vi "FPGA.vi"() -> ()   [LabVIEW 2013]
doc: "This is the primary FPGA VI for the Build Your Own Embedded System project."
uses:
  <vilib>/Platform/TimedLoop/XDataNode/timing_clust.ctl
  <vilib>/Platform/TimedLoop/XDataNode/nitl_modes.ctl
  <vilib>/Platform/TimedLoop/XDataNode/wakeup.ctl
  <vilib>/rvi/FXPMathLib/FxpDiv/subVIs/nifxpmath_Div_SimConfig.ctl
  <vilib>/rvi/Emulation/niFpgaSctlEmulationGetInTimedLoop.vi
  <vilib>/rvi/Emulation/niFpgaEmulationReportErrorSimple.vi
  <vilib>/rvi/Emulation/niFpgaGetClockAttributes.vi
  <vilib>/rvi/eio/common/nirviEmuTemplateMethod_errors.vi
  <vilib>/rvi/Emulation/niFpgaCriticalErrorInLSC.vi
  <vilib>/rvi/Analysis/utilities/niFPGA Threshold Crossing Logic.vi
  <vilib>/rvi/FXPMathLib/FxpDiv/simVIs/DllFxpDivTemp_sub.vi
  <vilib>/rvi/Analysis/measure/period/templates/niFPGA Period Edge Direction.ctl
  <vilib>/eio/EIONode/EIONode.xnode
  <vilib>/rvi/Analysis/measure/period/XNode/niFpgaAnalogPeriod.xnode
  <vilib>/Platform/TimedLoop/XDataNode/XDataNode.xnode
  <vilib>/rvi/FXPMathLib/FxpDiv/XNode/nifxpmath_Div.xnode
  <vilib>/rvi/Analysis/measure/butterworth/XNode/niFpgaButterworthFilter.xnode
  <vilib>/addons/control/pid/fpga.llb/XNode/niFpgaPID.xnode
  <vilib>/rvi/FXPMathLib/FxpInterpret/XNode/nifxpmath_Interpret.xnode
  <vilib>/Platform/TimedLoop/XDataNode/XDNodeRunTimeDep.lvlib
panel:
  in  "Invert Polarity?":bool=TRUE
  in  "stop bits (10: 1 bit)":u16(ring)=10 items=["1.0"=10, "1.5"=15, "2.0"=20]
  in  "data bits (8)":i32=8 min=5 max=8 step=1
  in  "parity (0:none)":enum16{"None", "Odd", "Even", "Mark", "Space"}(ring)
  in  "baud rate":u32=1200000
  out "PIDOut":fxp<+/-,16,8>
  in  "PIDSetpoint":fxp<+/-,16,18>
  in  "PID gains":T1={"proportional gain (Kc)"=1.0, "integral gain (Kc*Ts/Ti)"=0.015625, "derivative gain (Kc*Td/Ts)"=0.0}
  in  "CommandFilterCoeff":i32[](array[numeric])=[-955995012, 2025731616, 1001305, -1023351008, 2092954700, 1034533]
  in  "UsePID":bool
  in  "DeadCount":u32=100
  in  "JerkThresh":fxp<+/-,37,22>=100.0
  out "Jerk":fxp<+/-,37,22>
  out "Accel":fxp<+/-,33,18>
  out "Speed":fxp<+/-,33,18>
  out "State":enum16{"Forward", "Reverse"}(ring)
  out "FilteredRPM":fxp<+/-,33,18>
  out "Direction":bool
  in  "SpeedFilterCoeff":i32[](array[numeric])=[-955995012, 2025731616, 1001305, -1023351008, 2092954700, 1034533]
  out "SpeedCommandOut":fxp<+/-,23,8>
  in  "PeriodHysteresis":fxp<+,23,4>=0.5
  in  "PeriodThreshold":fxp<+/-,24,5>=2.0
  in  "SpeedCommand":fxp<+/-,20,5>
  in  "DriveEnable":bool
  out "Potentiometer":fxp<+/-,24,5>
  out "RPM":fxp<+,32,16>
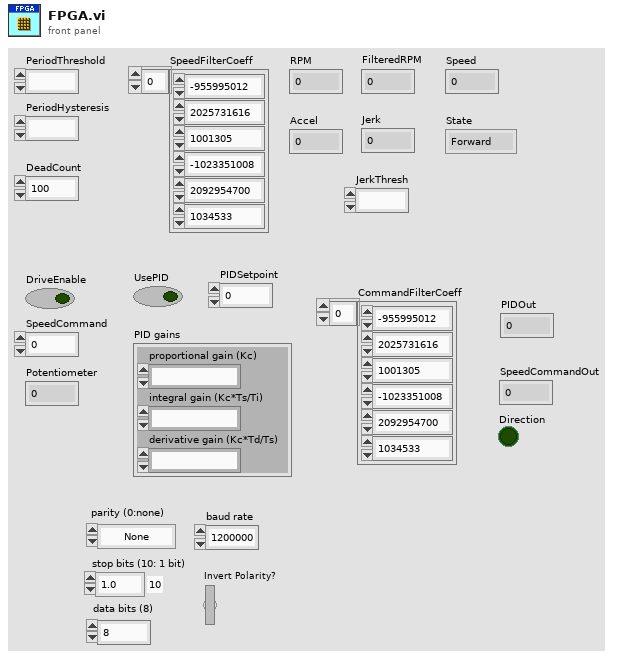
[diagram p1: front panel]
types:
  T1 = cluster{"proportional gain (Kc)":fxp<+/-,16,8>, "integral gain (Kc*Ts/Ti)":fxp<+/-,16,8>, "derivative gain (Kc*Td/Ts)":fxp<+/-,16,8>}
  T2 = typedef "XDNodeRunTimeDep.lvlib/timing_clust.ctl" = cluster{"Expected End [f-1]":u64, "Actual End [f-1]":u64, "Finished Late? [f-1]":bool, "Expected End [i-1]":u64, "Actual End [i-1]":u64, "Finished Late? [i-1]":bool, "Expected Start [i]":u64, "Actual Start [i]":u64, "Expected Start [f]":u64, "Actual Start [f]":u64, "Source Name":string, "Structure Name":string, "Period":i64, "Deadline":i64, "Offset":i64, "Start":i64, "Priority":i32, "Timeout":i32, "Mode":T3, "Wakeup Reason":T4, "Error":errorcluster, "Source Type":string, "Secondary Source Type":string, "Global End Time":u64, "Global Start Time":u64, "Frame Duration":u64, "Iteration Duration":u64, "Assigned CPU":i32, "I/O Scan Engine Mode":u32}
  T3 = typedef "XDNodeRunTimeDep.lvlib/nitl_modes.ctl" = enum32{"No Change", "Process missed periods, maintain original phase", "Discard missed periods, maintain original phase", "Process missed periods, ignore original phase", "Discard missed periods, ignore original phase"}
  T4 = typedef "XDNodeRunTimeDep.lvlib/wakeup.ctl" = enum32{"Normal", "Aborted", "Asynchronous wakeup", "Timing source error", "Timed loop error", "Timeout"}
  T5 = cluster{"proportional gain (Kc)":i16, "integral gain (Kc*Ts/Ti)":i16, "derivative gain (Kc*Td/Ts)":i16}
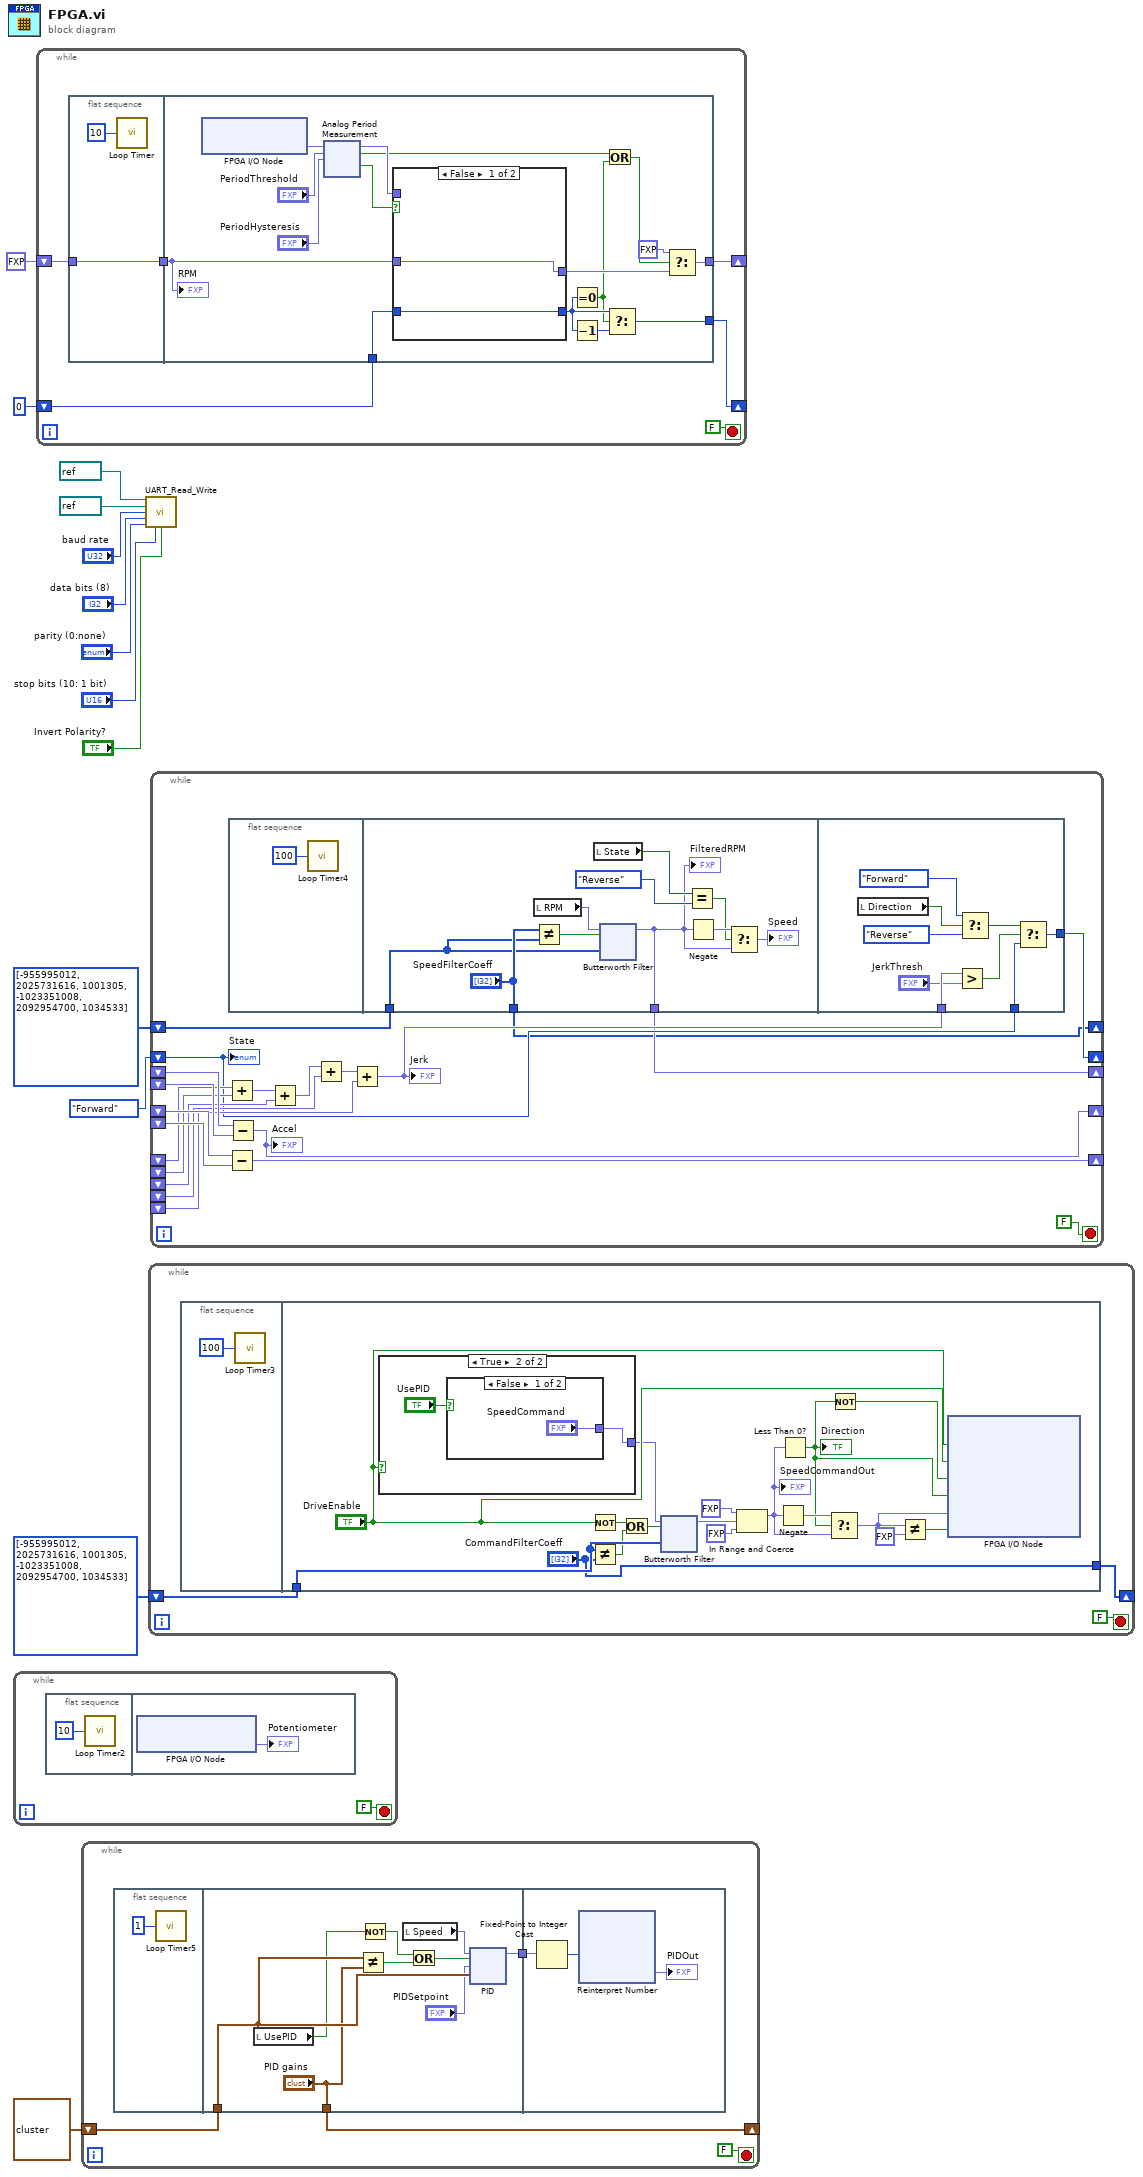
[diagram p0: block diagram]
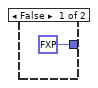
[diagram p2: hidden frame]
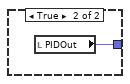
[diagram p3: hidden frame]
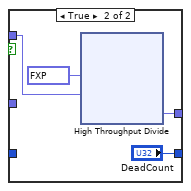
[diagram p4: hidden frame]
diagram:
  n1 = while {
    stop <- FALSE stop-if-true
    n2 = flat-sequence {
      frame #0 {
        n3 = call "Loop Timer2"("Count(mSec)"=u32 10 ("Count(uSec)")) -> ()  [unwired: 1 out]
      }
      frame #1 {
        n4 = xnode "FPGA I/O Node"() -> ("Potentiometer"=→"Potentiometer":fxp<+/-,24,5>)  [unwired: 1 in, 1 out]
      }
    }
  }
  n5 = while {
    shift-right: [w21] -> _
    shift-left: fxp<+,32,16> 0.0 ("x/y") -> [w20]
    shift-right: [w18] -> _
    shift-left: u32 0 ("DeadCount") -> [w17]
    stop <- FALSE stop-if-true
    n6 = flat-sequence {
      tunnel: w20 -> [w24]
      tunnel: [w24] -> w19
      tunnel: w19 -> [w31]
      tunnel: [w34] -> w21
      tunnel: [w27] -> w18
      tunnel: w17 -> [w32]
      frame #0 {
        n7 = call "Loop Timer"("Count(uSec)"=u32 10) -> ()  [unwired: 1 out]
      }
      frame #1 {
        n8 = xnode "FPGA I/O Node"() -> ("MotorPWM"=w40:fxp<+/-,24,5>)  [unwired: 1 in, 1 out]
        n9 = xnode "Analog Period Measurement"("input data"=w40, "threshold level"="PeriodThreshold", "hysteresis"="PeriodHysteresis") -> ("period (samples)"=w38:fxp<+,32,16>, "output valid"=w39:bool, "timeout"=w30:bool)  [unwired: 2 in, 1 out]
        n10 = case shown="False" w39 {
          tunnel: w38 -> [_ w46]
          tunnel: [w42 w44] -> w35
          tunnel: w31 -> [w42 _]
          tunnel: [w41 "DeadCount"] -> w28
          tunnel: w32 -> [w41 _]
          frame False {
          }
          frame True {
            n11 = xnode "High Throughput Divide"("x"=fxp<+,32,32> 100000.0, "y"=w46) -> ("x/y"=w44:fxp<+,32,16>)
          }
        }
        n12 = Equal To 0?(x=w28) -> (x = 0?=w25:bool)
        n13 = Decrement(x=w28) -> (x-1=w26:u32)
        n14 = Or(x=w30, y=w25) -> (x .or. y?=w29:bool)
        n15 = Select(t=w28, s=w25, f=w26) -> (s? t:f=w27:u32)
        n16 = Select(t=fxp<+,32,16> 0.0, s=w29, f=w35) -> (s? t:f=w34:fxp<+,32,16>)
        "RPM" <- w31
      }
    }
  }
  n17 = while {
    shift-right: [w192] -> _
    shift-left: T1 {"proportional gain (Kc)"=1.0, "integral gain (Kc*Ts/Ti)"=0.015625, "derivative gain (Kc*Td/Ts)"=0.0} ("PID gains") -> [w191]
    stop <- FALSE stop-if-true
    n18 = flat-sequence {
      tunnel: ["PID gains"] -> w192
      tunnel: w191 -> [w202]
      tunnel: [w194] -> w190
      tunnel: w190 -> [w233]
      frame #0 {
        n19 = call "Loop Timer5"("Count(mSec)"=u32 1 ("Count(uSec)")) -> ()  [unwired: 1 out]
      }
      frame #1 {
        n20 = local read "UsePID"() -> (w200:bool)
        n21 = Not Equal?(x=w202, y="PID gains") -> (x != y?=w198:bool)
        n22 = Not(x=w200) -> (.not. x?=w199:bool)
        n23 = local read "Speed"() -> (w196:fxp<+/-,33,18>)
        n24 = Or(x=w199, y=w198) -> (x .or. y?=w197:bool)
        n25 = xnode "PID"("process variable"=w196, "reset?"=w197, "setpoint"="PIDSetpoint", "PID gains"=w202) -> ("output"=w194:fxp<+/-,16,18>)  [unwired: 1 in]
      }
      frame #2 {
        n26 = Fixed-Point to Integer Cast(1:w233) -> (0:w232:i16)
        n27 = xnode "Reinterpret Number"("x"=w232) -> ("y"=→"PIDOut":fxp<+/-,16,8>)
      }
    }
  }
  n28 = call "UART_Read_Write.vi"("Transmit"=refnum<k21> "TX", "Receive"=refnum<k21> "RX", "baud rate (9600)"="baud rate", "data bits (8)"="data bits (8)", "parity (0:none)"="parity (0:none)", "stop bits (10: 1 bit)"="stop bits (10: 1 bit)", "Invert Polarity?"="Invert Polarity?") -> ()  [unwired: 9 in]
  n29 = while {
    shift-right: [w235] -> _
    shift-left: i32[] [-955995012, 2025731616, 1001305, -1023351008, 2092954700, 1034533] ("CommandFilterCoeff") -> [w234]
    stop <- FALSE stop-if-true
    n30 = flat-sequence {
      tunnel: ["CommandFilterCoeff"] -> w235
      tunnel: w234 -> [w245]
      frame #0 {
        n31 = call "Loop Timer3"("Count(uSec)"=u32 100) -> ()  [unwired: 1 out]
      }
      frame #1 {
        n32 = case shown="True" "DriveEnable" {
          tunnel: [fxp<+/-,20,5> 0.0 ("SpeedCommand") w265] -> w240
          frame False {
          }
          frame True {
            n33 = case shown="False" "UsePID" {
              tunnel: ["SpeedCommand" w267] -> w265
              frame False {
              }
              frame True {
                n34 = local read "PIDOut"() -> (w267:fxp<+/-,16,8>)
              }
            }
          }
        }
        n35 = Not(x="DriveEnable") -> (.not. x?=w243:bool)
        n36 = Not Equal?(x=w245, y="CommandFilterCoeff") -> (x != y?=w242:bool)
        n37 = Or(x=w243, y=w242) -> (x .or. y?=w241:bool)
        n38 = xnode "Butterworth Filter"("input data"=w240, "reset"=w241, "scaled coefficients"=w245) -> ("output data"=w239:fxp<+/-,23,8>)
        n39 = In Range and Coerce(upper limit=fxp<+/-,20,5> 5.0, x=w239, lower limit=fxp<+/-,20,5> -5.0) -> (coerced(x)=w238:fxp<+/-,23,8>)  [unwired: 1 out]
        "SpeedCommandOut" <- w238
        n40 = Negate(x=w238) -> (-x=w251:fxp<+/-,20,5>)
        n41 = Less Than 0?(x=w238) -> (x < 0?=w247:bool)
        "Direction" <- w247
        n42 = Select(t=w251, s=w247, f=w238) -> (s? t:f=w250:fxp<+/-,23,8>)
        n43 = Not(x=w247) -> (.not. x?=w252:bool)
        n44 = Not Equal?(x=w250, y=fxp<+/-,20,5> 0.0) -> (x != y?=w253:bool)
        n45 = xnode "FPGA I/O Node"("EnableOut"="DriveEnable", "Enable"="DriveEnable", "DirectionOut"=w252, "Direction"=w247, "SpeedCommand"=w250, "Running"=w253) -> ()  [unwired: 6 in, 6 out]
      }
    }
  }
  n46 = while {
    shift-right: [w270] -> _
    shift-left: _ -> [w287]
    shift-right: [w271] -> _
    shift-left: enum16{"Forward", "Reverse"}."Forward" -> [w272]
    shift-left: _ -> [w286]
    shift-right: [w285] -> _
    shift-left: _ -> [w284]
    shift-left: _ -> [w283]
    shift-right: [w282] -> _
    shift-left: _ -> [w281]
    shift-left: _ -> [w280]
    shift-left: _ -> [w278]
    shift-left: _ -> [w276]
    shift-left: _ -> [w274]
    shift-right: [w269] -> _
    shift-left: i32[] [-955995012, 2025731616, 1001305, -1023351008, 2092954700, 1034533] ("FilterCoeff") -> [w268]
    stop <- FALSE stop-if-true
    n47 = Add(x=w281, y=w280) -> (x+y=w279:fxp<+/-,35,20>)
    n48 = Subtract(x=w284, y=w283) -> (x-y=w282:fxp<+/-,34,19>)
    n49 = Subtract(x=w287, y=w286) -> (x-y=w285:fxp<+/-,33,18>)
    "Accel" <- w285
    n50 = flat-sequence {
      tunnel: [w293] -> w270
      tunnel: ["SpeedFilterCoeff"] -> w269
      tunnel: w268 -> [w291]
      tunnel: w273 -> [w316]
      tunnel: w272 -> [w313]
      tunnel: [w312] -> w271
      frame #0 {
        n51 = call "Loop Timer4"("Count(uSec)"=u32 100) -> ()  [unwired: 1 out]
      }
      frame #1 {
        n52 = local read "RPM"() -> (w299:fxp<+,32,16>)
        n53 = Not Equal?(x="SpeedFilterCoeff", y=w291) -> (x != y?=w290:bool)
        n54 = local read "State"() -> (w296:enum16{"Forward", "Reverse"})
        n55 = xnode "Butterworth Filter"("input data"=w299, "reset"=w290, "scaled coefficients"=w291) -> ("output data"=w293:fxp<+/-,32,17>)
        "FilteredRPM" <- w293
        n56 = Equal?(x=w296, y=enum16{"Forward", "Reverse"}."Reverse") -> (x = y?=w297:bool)
        n57 = Negate(x=w293) -> (-x=w298:fxp<+/-,33,18>)
        n58 = Select(t=w298, s=w297, f=w293) -> (s? t:f=→"Speed":fxp<+/-,33,18>)
      }
      frame #2 {
        n59 = local read "Direction"() -> (w311:bool)
        n60 = Greater?(x=w316, y="JerkThresh") -> (0:w314:bool)
        n61 = Select(t=enum16{"Forward", "Reverse"}."Forward" ("y"), s=w311, f=enum16{"Forward", "Reverse"}."Reverse" ("y")) -> (s? t:f=w308:enum16{"Forward", "Reverse"})
        n62 = Select(t=w308, s=w314, f=w313) -> (s? t:f=w312:enum16{"Forward", "Reverse"})
      }
    }
    n63 = Add(x=w279, y=w278) -> (x+y=w277:fxp<+/-,36,21>)
    n64 = Add(x=w277, y=w276) -> (x+y=w275:fxp<+/-,36,21>)
    n65 = Add(x=w275, y=w274) -> (x+y=w273:fxp<+/-,37,22>)
    "Jerk" <- w273
    "State" <- w272
  }
